vi "KE622x -- DCon Mode Get 2182 -A Present State.vi"(0 "Resource In":refnum<visa-resource-name>, 1 "Check For SCPI Errors? (T)":bool=TRUE, 11 "error in (no error)":errorcluster) -> (4 "Resource Out (dupl)":refnum<visa-resource-name>, 8 "2182/2182A Present?":bool, 15 "error out":errorcluster)   [LabVIEW 2019, in "Keithley 622x.lvlib"]
uses:
  Keithley 622x.lvlib
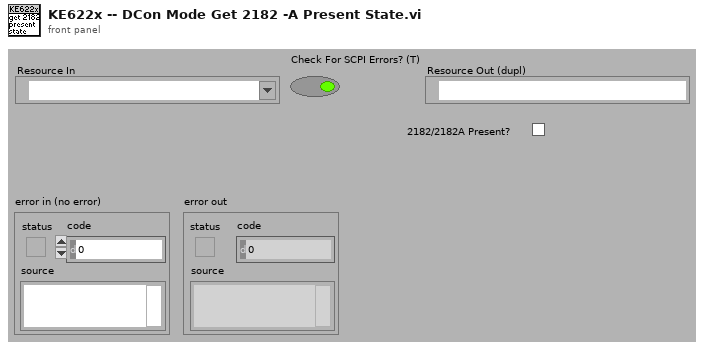
[diagram p1: front panel]
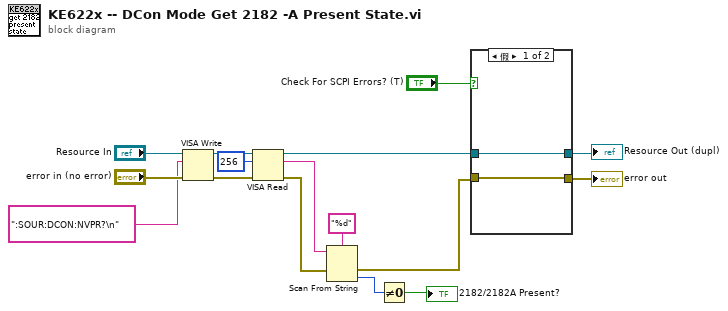
[diagram p0: block diagram]
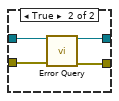
[diagram p2: hidden frame]
diagram:
  n1 = VISA Write(VISA resource name="Resource In", write buffer=":SOUR:DCON:NVPR?\n" ("format string"), error in (no error)="error in (no error)") -> (VISA resource name out=w11:refnum<visa-resource-name>, error out=w10:errorcluster)  [unwired: 1 out]
  n2 = VISA Read(VISA resource name=w11, byte count=u32 256, error in (no error)=w10) -> (VISA resource name out=w4:refnum<visa-resource-name>, read buffer=w6:string, error out=w8:errorcluster)  [unwired: 1 out]
  n3 = Scan From String(format string="%d", input string=w6, error in=w8) -> (error out=w5:errorcluster, output 1=w2:i32)  [unwired: 2 in, 2 out]
  n4 = Not Equal To 0?(x=w2) -> (x != 0?=→"2182/2182A Present?":bool)
  n5 = case shown="假" "Check For SCPI Errors? (T)" {
    tunnel: w4 -> [w18 w22]
    tunnel: w5 -> [w17 w21]
    tunnel: [w17 w20] -> w12
    tunnel: [w18 w19] -> w13
    frame False {
    }
    frame True {
      n6 = call "Error Query.vi"("VISA Resource In"=w22, "error in (no error)"=w21) -> ("VISA Resource Out (dupl)"=w19:refnum<visa-resource-name>, "error out"=w20:errorcluster)  [unwired: 10 in, 2 out]
    }
  }
  "Resource Out (dupl)" <- w13
  "error out" <- w12
